vi "Initialize.vi"(8 "error in":errorcluster, 10 "shared resources":refnum<class "Shared Resources.lvclass">, 11 "Tx Execution Unit Implementation in":refnum<class "Tx Generic Execution Unit.lvclass">) -> (0 "error out":errorcluster, 3 "Tx Execution Unit Implementation out":refnum<class "Tx Generic Execution Unit.lvclass">)   [LabVIEW 2020, in "AIM ARINC 664 Engine.lvlib" / "Implementation.lvlib" / "Tx Generic Execution Unit.lvclass"]
uses:
  Tx Generic Execution Unit.lvclass
  Tx Generic Execution Unit.lvclass/Tx Generic Execution Unit.ctl
  <instrlib>/AIM GmbH/_AIM 664/AIM664LV.lvlib
  <vilib>/Utility/SystemLogging/NI_SystemLogging.lvlib
  <instrlib>/AIM GmbH/_AIM 664/bsp/Fdx Create Session (Tx-Generic).vi
  Interfaces/Shared Resources/Shared Resources.lvclass
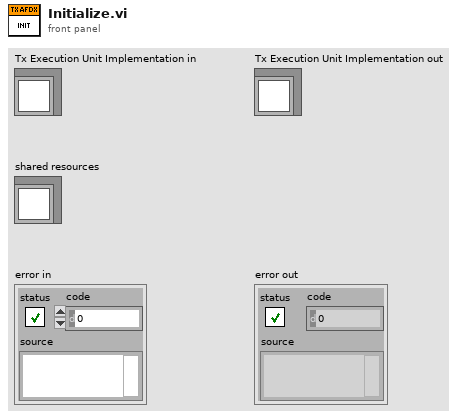
[diagram p1: front panel]
types:
  T1 = typedef "channel_settings_tx.ctl" = cluster{"Tx Board":u32, "Tx Port":u32, "Payload Parameter Array":T2[], "QueueSizeIn":u32, "Count":u32, "StartMode":u32}
  T2 = typedef "Frame Payload Parameters.ctl" = cluster{"PayloadID":string, "FrameIndeces":u32[], "Parameters":cluster{"start index":i32, "size":i32, "encoding":T3, "signed":bool, "scale multiplier":dbl, "scale offset":dbl}[]}
  T3 = typedef "Encoding (Arinc664).ctl" = u16
  T4 = typedef "RawFrame_entry.ctl" = cluster{"HeaderInfo":T5, "PayloadID":string}
  T5 = typedef "AIM664LV.lvlib/queue_header_generic.ctl" = cluster{"InterFrameGap":u32, "PacketGroupWaitTime":u32, "PayloadBufferMode":u8, "PayloadGenerationMode":u8, "PreambleCount":u8, "Skew":u32, "NetSelect":u8, "FrameStartMode":u8, "PhysErrorInjection":u32, "SequenceNumberInit":u16, "SequenceNumberOffset":u16}
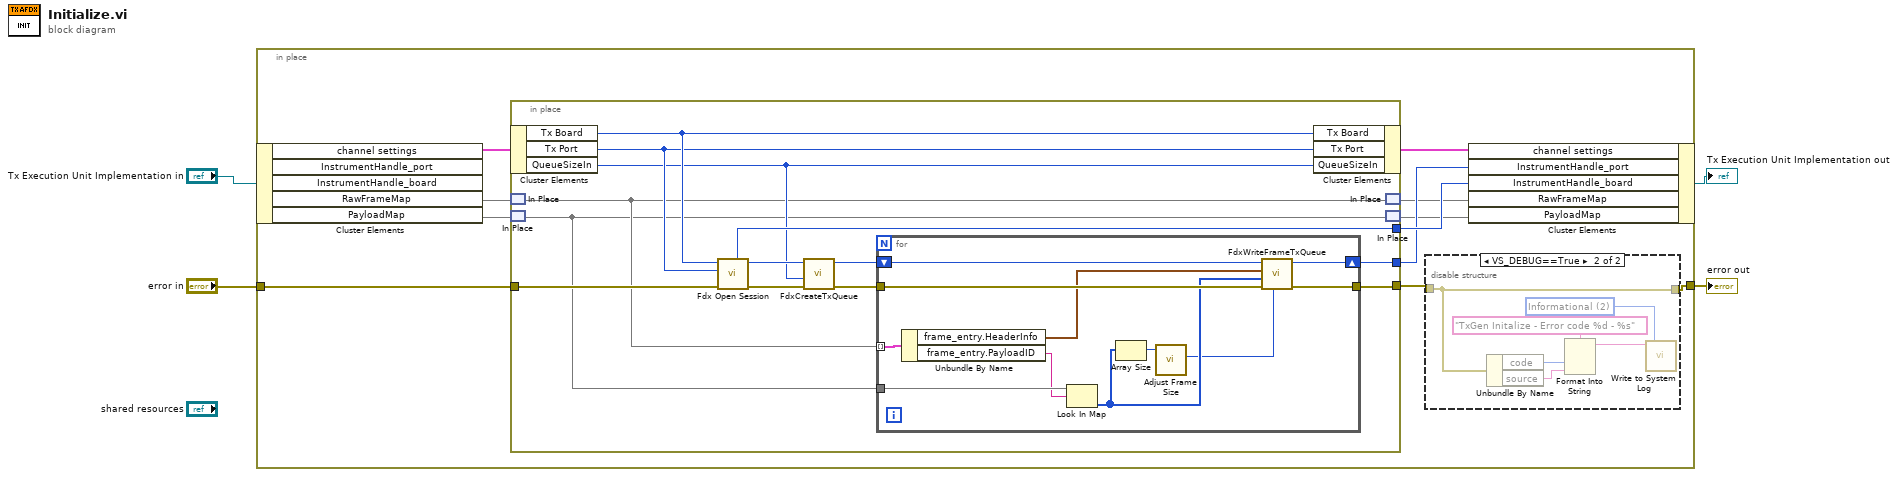
[diagram p0: block diagram]
diagram:
  n1 = in-place {
    in-place-border: "error in" -> [w15]
    in-place-border: [w9] -> w1
    n2 = in-place-cluster #1("Tx Execution Unit Implementation in") -> ("channel settings"=w14:T1, "RawFrameMap"=w8:map{string, T4}, "PayloadMap"=w7:map{string, u8[]})  [unwired: 2 out]
    n3 = in-place {
      in-place-border: w15 -> [w25]
      in-place-border: [w28] -> w12
      in-place-border: [w26] -> w11
      in-place-border: [w19] -> w10
      n4 = in-place-cluster #2(w14) -> ("Tx Board"=w23:u32, "Tx Port"=w22:u32, "QueueSizeIn"=w18:u32)
      n5 = in-place-match #3(w8) -> (w17:map{string, T4})
      n6 = in-place-match #4(w7) -> (w16:map{string, u8[]})
      n7 = call-poly <instrlib>:"Fdx Open Session.vi"("error in (no error)"=w25, "port"=w22, "board"=w23) -> ("error out"=w21:errorcluster, "port handle out"=w24:u32, "InstrumentHandle_board out"=w28:u32)  [unwired: 3 in, 3 out]
      n8 = call <instrlib>:"FdxCreateTxQueue.vi"("error in"=w21, "QueueSizeIn"=w18, "InstrumentHandle_port"=w24) -> ("error out"=w20:errorcluster, "InstrumentHandle_port"=w27:u32)  [unwired: 6 in, 1 out]
      n9 = for {
        tunnel: w20 -> [w37]
        tunnel: [w36] -> w19
        shift-right: [w38] -> w26
        shift-left: w27 -> [w39]
        tunnel: w17 -> [w35] mode=indexing
        tunnel: w16 -> [w34]
        n10 = Unbundle By Name(w35) -> ("frame_entry.HeaderInfo"=w32:T5, "frame_entry.PayloadID"=w33:string)
        n11 = Look In Map(map=w34, key=w33) -> (value=w31:u8[])  [unwired: 1 in, 1 out]
        n12 = Array Size(array=w31) -> (size(s)=w30:i32)
        n13 = call "Adjust Frame Size.vi"("original size in"=w30) -> ("adjusted size"=w29:i32)  [unwired: 8 in, 2 out]
        n14 = call <instrlib>:"FdxWriteFrameTxQueue.vi"("Frame Size"=w29, "error in (no error)"=w37, "Frame in"=w31, "HeaderInfo"=w32, "InstrumentHandle_port in"=w39) -> ("error out"=w36:errorcluster, "InstrumentHandle_port out"=w38:u32)  [unwired: 5 in]
      }
      n15 = in-place-cluster #2("Tx Board"=w23, "Tx Port"=w22, "QueueSizeIn"=w18) -> (w13:T1)
      n16 = in-place-match #3(w17) -> (w6:map{string, T4})
      n17 = in-place-match #4(w16) -> (w5:map{string, u8[]})
    }
    n18 = disable-structure shown="VS_DEBUG==True" {
      disable-tunnel: w10 -> [w40 w41]
      disable-tunnel: [w40 w41] -> w9
      frame condition #0 (active) {
      }
      frame condition #1 {
        w44 = 2 items=["Error", "Warning", "Informational"] ("severity")
        n19 = Unbundle By Name(w41) -> ("code"=w43:i32, "source"=w42:string)
        n20 = Format Into String(format string="TxGen Initalize - Error code %d - %s", w43, w42) -> (resulting string=w45:string)  [unwired: 2 in, 1 out]
        n21 = call <vilib>:"Write to System Log.vi"("severity"=w44, "message"=w45) -> ()  [unwired: 9 in, 1 out]
      }
    }
    n22 = in-place-cluster #1("channel settings"=w13, "InstrumentHandle_port"=w11, "InstrumentHandle_board"=w12, "RawFrameMap"=w6, "PayloadMap"=w5) -> (→"Tx Execution Unit Implementation out":refnum<class "Tx Generic Execution Unit.lvclass">)
  }
  "error out" <- w1
